vi "tsdb_get_flexray_signal_properties_by_index_verbose.vi"(8 "error in (no error)":errorcluster caption="错误输入（无错误）", 10 "ADBIndex":i32, 11 "path in":path) -> (0 "error out":errorcluster caption="错误输出", 1 "flexray_signal_properties_by_index":T1 {"ACompuMethod" items=["fcmIdentical", "fcmLinear", "fcmScaleLinear", "fcmTextTable", "fcmTABNoIntp", "fcmFormula"]; "ASignalType" items=["stCANSignal", "stLINSignal", "stSystemVar", "stFlexRay", "stEthernet"]}, 2 "function return":i32, 3 "path out":path)   [LabVIEW 2014]
doc: "TSAPI(s32)tsdb_get_flexray_signal_properties_by_index_verbose(const s32 ADBIndex,const s32 AECUIndex,const s32 AFrameIndex,const s32 ASignalIndex,const bool AIsTx,TSignalType* ASignalType,TFlexRayCompuMethod* ACompuMethod,bool* AIsIntel,s32* AActualStartBit,s32* AActualUpdateBit,s32* ALength,double* AFactor,double* AOffset,double* AInitValue,const ppchar AName,const ppchar AComment);"
uses:
  Typedef/FlexRay/flexray_signal_properties_by_index.ctl
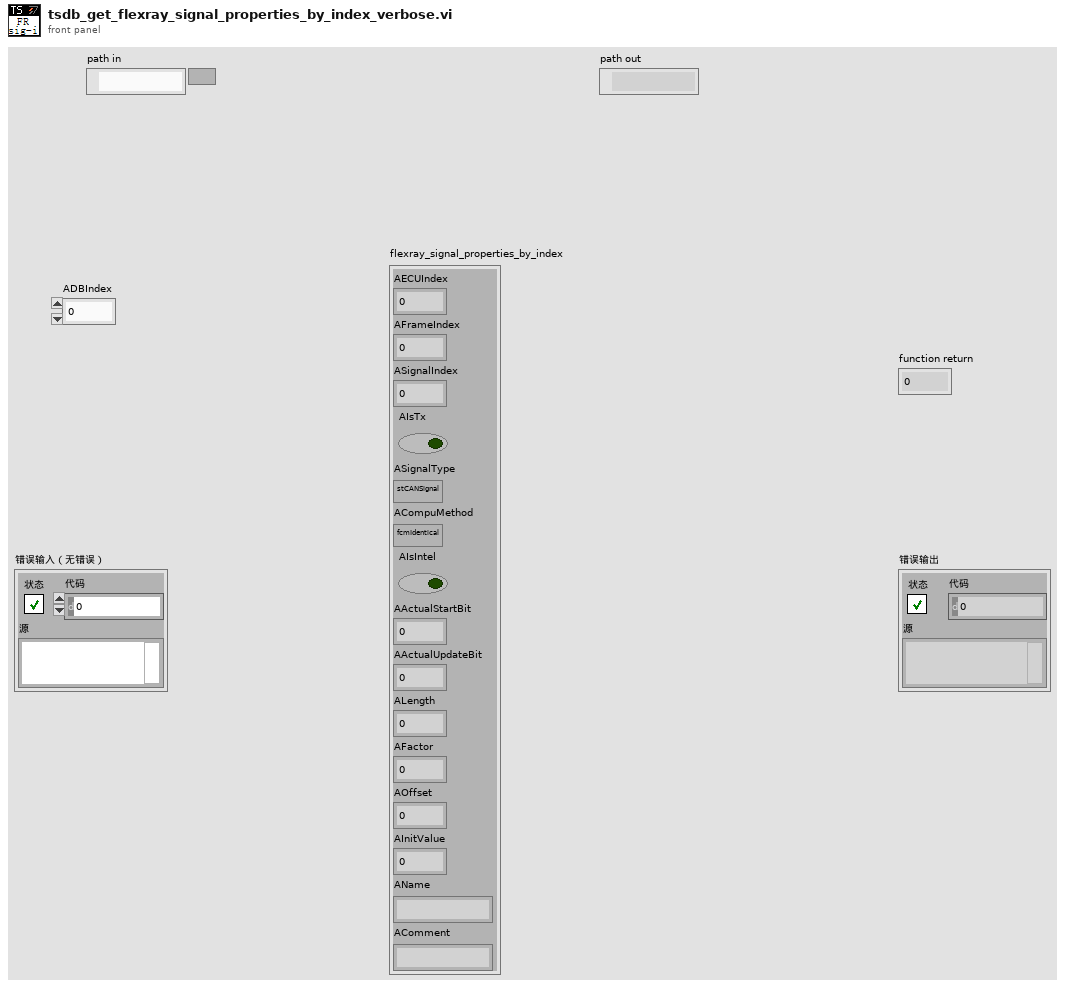
[diagram p1: front panel]
types:
  T1 = typedef "flexray_signal_properties_by_index.ctl" = cluster{"AECUIndex":i32, "AFrameIndex":i32, "ASignalIndex":i32, "AIsTx":bool, "ASignalType":u32, "ACompuMethod":u32, "AIsIntel":bool, "AActualStartBit":i32, "AActualUpdateBit":i32, "ALength":i32, "AFactor":dbl, "AOffset":dbl, "AInitValue":dbl, "AName":string, "AComment":string}
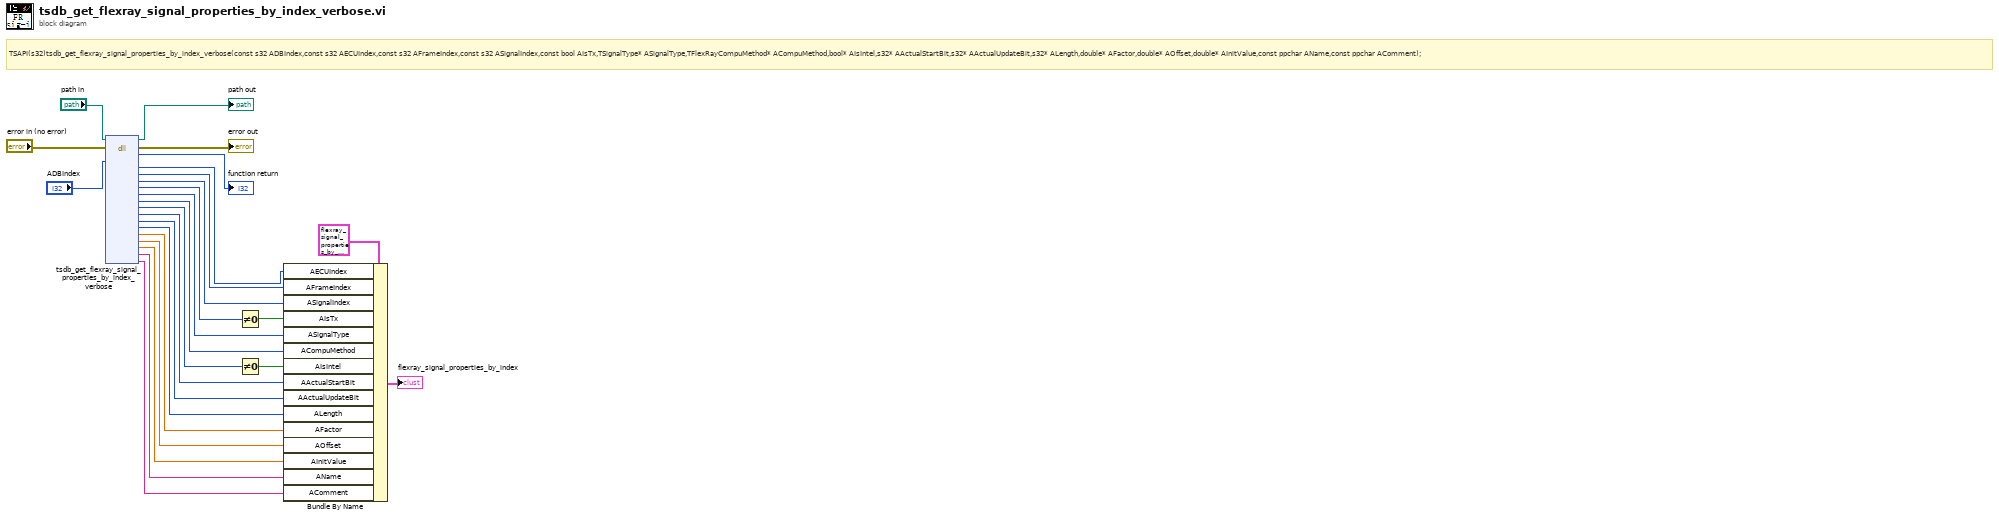
[diagram p0: block diagram]
diagram:
  # "TSAPI(s32)tsdb_get_flexray_signal_properties_by_index_verbose(const s32 ADBIndex,const s32 AECUIndex,const s32 AFrameIndex,const s32 ASignalIndex,const bool AIsTx,TSignalType* ASignalType,TFlexRayCompuMethod* ACompuMethod,bool* AIsIntel,s32* AActualStartBit,s32* AActualUpdateBit,s32* ALength,double* AFactor,double* AOffset,double* AInitValue,const ppchar AName,const ppchar AComment);"
  n1 = dll-call lib="D:/Work/LabVIEW Code/TSMaster Labview SDK/LabVIEW/LabVIEW-TSMasterAPI_CLN/TSMasterAPI_LabVIEW-2024-10-08 14-20-13/Not_organized_vi/TSMaster.*" fn="tsdb_get_flexray_signal_properties_by_index_verbose"(path in="path in", error in="error in (no error)", "ADBIndex"="ADBIndex") -> (path out=→"path out":path, error out=→"error out":errorcluster, "返回类型"=→"function return":i32, "AECUIndex"=w17:i32, "AFrameIndex"=w16:i32, "ASignalIndex"=w15:i32, "AIsTx"=w2:u8, "ASignalType"=w14:u32, "ACompuMethod"=w13:u32, "AIsIntel"=w1:u8, "AActualStartBit"=w12:i32, "AActualUpdateBit"=w11:i32, "ALength"=w10:i32, "AFactor"=w9:dbl, "AOffset"=w8:dbl, "AInitValue"=w7:dbl, "AName"=w6:string, "AComment"=w5:string)  [unwired: 17 in]
  n2 = Not Equal To 0?(x=w2) -> (x != 0?=w3:bool)
  n3 = Not Equal To 0?(x=w1) -> (x != 0?=w4:bool)
  n4 = Bundle By Name(cluster=T1 {"AECUIndex"=0, "AFrameIndex"=0, "ASignalIndex"=0, "AIsTx"=FALSE, "ASignalType"=0, "ACompuMethod"=0, "AIsIntel"=FALSE, "AActualStartBit"=0, "AActualUpdateBit"=0, "ALength"=0, "AFactor"=0.0, "AOffset"=0.0, "AInitValue"=0.0, "AName"="", "AComment"=""} ("flexray_signal_properties_by_index"), "AECUIndex"=w17, "AFrameIndex"=w16, "ASignalIndex"=w15, "AIsTx"=w3, "ASignalType"=w14, "ACompuMethod"=w13, "AIsIntel"=w4, "AActualStartBit"=w12, "AActualUpdateBit"=w11, "ALength"=w10, "AFactor"=w9, "AOffset"=w8, "AInitValue"=w7, "AName"=w6, "AComment"=w5) -> (→"flexray_signal_properties_by_index":T1)
